vi "Write Instrument Handle.vi"(8 "error in (no error)":errorcluster, 10 "Resource name":refnum<k15>="AGILENT1", 11 "Agilent DSO-X 3032A in":refnum<class "Agilent DSO-X 3032A.lvclass">) -> (0 "error out":errorcluster, 3 "Agilent DSO-X 3032A out":refnum<class "Agilent DSO-X 3032A.lvclass">)   [LabVIEW 2014, in "Agilent DSO-X 3032A.lvclass"]
uses:
  Agilent DSO-X 3032A.lvclass
  Agilent DSO-X 3032A.lvclass/Agilent DSO-X 3032A.ctl
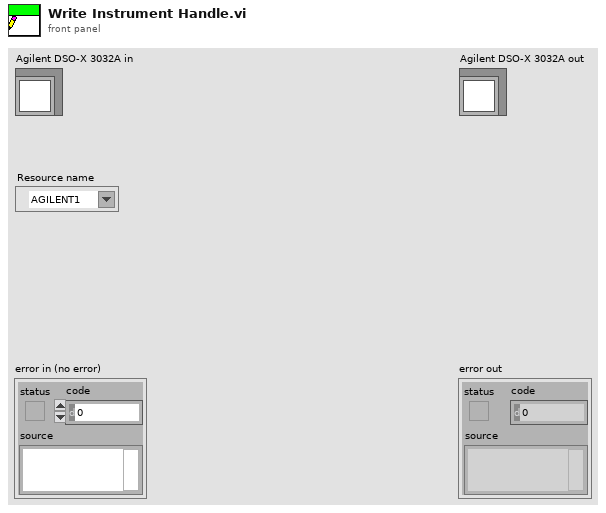
[diagram p1: front panel]
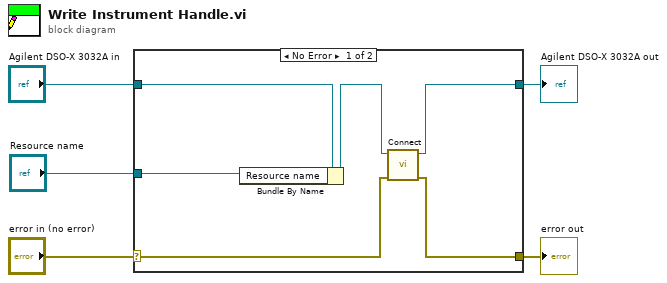
[diagram p0: block diagram]
diagram:
  n1 = case shown="No Error" "error in (no error)" {
    selector: "error in (no error)" -> [w8 w12]
    tunnel: [w7 w12] -> w4
    tunnel: [w9 w13] -> w2
    tunnel: "Agilent DSO-X 3032A in" -> [w11 w13]
    tunnel: "Resource name" -> [w6 _]
    frame No Error {
      n2 = Bundle By Name(cluster=w11, "Resource name"=w6) -> (w10:refnum<class "Agilent DSO-X 3032A.lvclass">)
      n3 = call-dynamic "Connect.vi"("error in (no error)"=w8, "Agilent DSO-X 3032A in"=w10) -> ("error out"=w7:errorcluster, "Agilent DSO-X 3032A out"=w9:refnum<class "Agilent DSO-X 3032A.lvclass">)  [unwired: 8 in]
    }
    frame Error {
    }
  }
  "error out" <- w4
  "Agilent DSO-X 3032A out" <- w2
